vi "S256 Code Challenge.vi"(10 "Code Verifier":string) -> (2 "Code Challenge":string)   [LabVIEW 2020, in "OAuth2.lvlib"]
doc: "Generates a S256 Code Challenge. This should be from a randomly generated string and is used to prevent CSRF authentication attacks during an authentication request. Unless implementing new authorization flows, this VI is not needed by external code."
uses:
  OAuth2.lvlib
  <vilib>/IlluminatedG/lv-web-crypto/lv-crypto/Crypto/Hashes/SHA-256/SHA-256.lvclass
  <vilib>/IlluminatedG/lv-web-crypto/lv-base64/Base64.lvlib
  <vilib>/IlluminatedG/lv-web-crypto/lv-base64/Variant.ctl
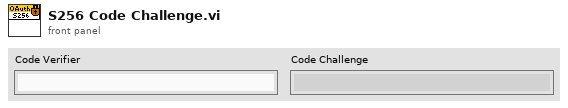
[diagram p1: front panel]
types:
  T1 = typedef "Base64.lvlib/Variant.ctl" = enum16{"Base64", "Base64-URL"}
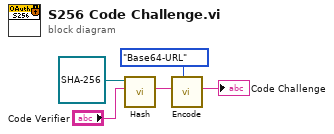
[diagram p0: block diagram]
diagram:
  n1 = call-dynamic "Hash.vi"("Message"="Code Verifier", "SHA-256 in"=refnum<class "SHA-256.lvclass"> refnum ("Crypto.lvlib:SHA-256.lvclass")) -> ("Hash"=w3:string)  [unwired: 7 in, 2 out]
  n2 = call <vilib>:"Encode.vi"("Variant (Base64)"=Variant."Base64-URL", "string in (not encoded)"=w3) -> ("string out (base64-encoded)"=→"Code Challenge":string)  [unwired: 8 in, 1 out]
